vi "start_stop.vi"(8 "error in (no error)":errorcluster, 10 "start? (T)":bool=TRUE, 11 "timer in":refnum<class "rytimer.lvclass">) -> (0 "error out":errorcluster, 3 "timer out":refnum<class "rytimer.lvclass">)   [LabVIEW 2017, in "rytimer.lvclass"]
uses:
  rytimer.lvclass
  rytimer.lvclass/rytimer.ctl
  state.ctl
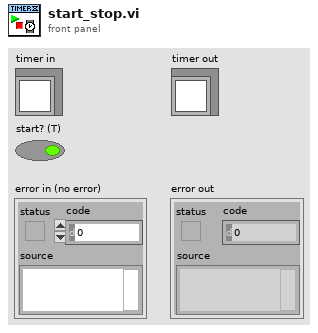
[diagram p1: front panel]
types:
  T1 = typedef "rytimer.lvclass/state.ctl" = enum8{"stop", "start", "mode", "interval", "message"}
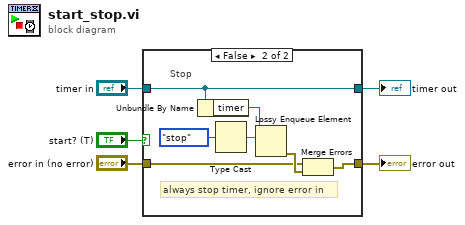
[diagram p0: block diagram]
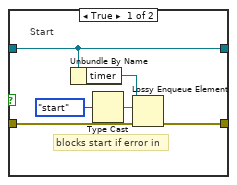
[diagram p2: hidden frame]
diagram:
  n1 = case shown="False" "start? (T)" {
    tunnel: [w11 w15] -> w3
    tunnel: "error in (no error)" -> [w9 w14]
    tunnel: "timer in" -> [w6 w13]
    tunnel: [w6 w13] -> w1
    frame True {
      # "Start"
      # "blocks start if error in"
      n2 = Unbundle By Name(w6) -> ("timer"=w7:refnum<queue>)
      n3 = Type Cast(x=state."start" ("state")) -> (*(type *) &x=w10:string)  [unwired: 1 in]
      n4 = Lossy Enqueue Element(queue=w7, element=w10, error in (no error)=w9) -> (error out=w11:errorcluster)  [unwired: 3 out]
    }
    frame False {
      # "always stop timer, ignore error in"
      # "Stop"
      n5 = Unbundle By Name(w13) -> ("timer"=w12:refnum<queue>)
      n6 = Type Cast(x=state."stop" ("state")) -> (*(type *) &x=w17:string)  [unwired: 1 in]
      n7 = Lossy Enqueue Element(queue=w12, element=w17) -> (error out=w18:errorcluster)  [unwired: 1 in, 3 out]
      n8 = Merge Errors(w14, w18) -> (w15:errorcluster)
    }
  }
  "error out" <- w3
  "timer out" <- w1
